vi "Begin.vi"(8 "error in":errorcluster) -> (0 "error out":errorcluster)   [LabVIEW 2015]
doc: "Called before other user functions, this VI is expected to open initial I/O refnums, load in file data, and do all program initialization. Notice that the <B>error out</B> terminal is simply used for data flow. Wiring it to other structures or subVIs ensures that this VI runs first."
uses:
  <vilib>/Rock Robotics/WPI/SafetyOutput/WPI_SafetyOutputConfigMenu.ctl
  <vilib>/Rock Robotics/WPI/DriverStation/WPI_DriverStationRobotMode2.ctl
  <vilib>/Rock Robotics/WPI/Joystick/WPI_JoystickDeviceEnum.ctl
  <vilib>/Rock Robotics/SystemInterfaces/DIO/FPGA_DIOChannel.ctl
  <vilib>/Rock Robotics/SystemInterfaces/DIO/FPGA_DIORelayChannel.ctl
  <vilib>/Rock Robotics/WPI/Solenoid/WPI_SolenoidChannel.ctl
  <vilib>/Rock Robotics/SystemInterfaces/DIO/FPGA_DIOPWMChannel.ctl
  <vilib>/Rock Robotics/SystemInterfaces/spilib/spi_bus.ctl
  Robot Global Data.vi
  <vilib>/Rock Robotics/Network Tables/NT Write String Array.vi
  <vilib>/Rock Robotics/WPI/Switch/WPI_SwitchOpenLimit.vi
  <vilib>/Rock Robotics/WPI/Solenoid/WPI_SolenoidOpenDouble.vi
  <vilib>/Rock Robotics/WPI/Counter/WPI_CounterDigitalInputToDigitalSource.vi
  <vilib>/Rock Robotics/WPI/MotorControl/WPI_MotorControlOpen VictorSP.vi
  <vilib>/Rock Robotics/WPI/MotorControl/WPI_MotorControlOpenCANTalonSRX.vi
  <vilib>/Rock Robotics/WPI/RobotDrive/WPI_RobotDriveOpen4MotorWithExistingMotors.vi
  <vilib>/Rock Robotics/WPI/Gyro/WPI_GyroXRS450_SPI_Open.vi
  <vilib>/Rock Robotics/WPI/Utilities/WPI_GetSetVariantRefNum.vi
  <vilib>/Rock Robotics/WPI/Accelerometer/InternalAccelerometer/WPI_AccelerometerInternalOpen.vi
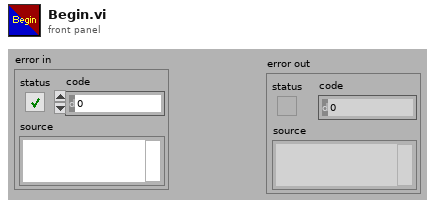
[diagram p1: front panel]
types:
  T1 = typedef "spi_bus.ctl" = enum16{"SPI On-Board, CS0", "SPI On-Board, CS1", "SPI On-Board, CS2", "SPI On-Board, CS3", "SPI MXP", "Invalid"}
  T2 = typedef "FPGA_DIOPWMChannel.ctl" = enum8{"PWM 0", "PWM 1", "PWM 2", "PWM 3", "PWM 4", "PWM 5", "PWM 6", "PWM 7", "PWM 8", "PWM 9", "PWM MXP 0", "PWM MXP 1", "PWM MXP 2", "PWM MXP 3", "PWM MXP 4", "PWM MXP 5", "PWM MXP 6", "PWM MXP 7", "PWM MXP 8", "PWM MXP 9", "Invalid"}
  T3 = typedef "FPGA_DIOChannel.ctl" = enum8{"DIO 0", "DIO 1", "DIO 2", "DIO 3", "DIO 4", "DIO 5", "DIO 6", "DIO 7", "DIO 8", "DIO 9", "DIO MXP 0", "DIO MXP 1", "DIO MXP 2", "DIO MXP 3", "DIO MXP 4", "DIO MXP 5", "DIO MXP 6", "DIO MXP 7", "DIO MXP 8", "DIO MXP 9", "DIO MXP 10", "DIO MXP 11", "DIO MXP 12", "DIO MXP 13", "DIO MXP 14", "DIO MXP 15", "Invalid"}
  T4 = typedef "WPI_SolenoidChannel.ctl" = enum8{"Solenoid 0", "Solenoid 1", "Solenoid 2", "Solenoid 3", "Solenoid 4", "Solenoid 5", "Solenoid 6", "Solenoid 7", "Invalid"}
  T5 = typedef "FPGA_DIORelayChannel.ctl" = enum8{"Relay 0", "Relay 1", "Relay 2", "Relay 3", "Invalid"}
  T6 = typedef "WPI_JoystickDeviceEnum.ctl" = enum16{"USB 0", "USB 1", "USB 2", "USB 3", "USB 4", "USB 5"}
  T7 = typedef "WPI_DriverStationRobotMode2.ctl" = enum16{"Autonomous Disabled", "Autonomous Enabled", "Teleop Disabled", "Teleop Enabled", "Disconnected", "Finish", "Test Disabled", "Test Enabled", "Emergency Stopped"}
  T8 = typedef "WPI_SafetyOutputConfigMenu.ctl" = enum16{"Enable", "Disable"}
  T9 = typedef "WPI_ServoDeviceRef.ctl" = cluster{"DeviceStatus":errorcluster, "PWM Channel":T2, "DeadBand":T10}
  T10 = typedef "WPI_PWMDeadband.ctl" = cluster{"Name":string, "maxPositivePwm":i32, "minPositivePwm":i32, "centerPwm":i32, "maxNegativePwm":i32, "minNegativePwm":i32, "angularRange":u16}
  T11 = typedef "WPI_MotorControlDeviceRef.ctl" = cluster{"DeviceStatus":errorcluster, "Type":T12, "PWM":cluster{"PWM Channel":T2, "DeadBand":T10}, "CAN":cluster{"Device Number":u8, "Control Mode":T13, "Semaphore":T14, "Max Vout":dbl, "TalonSRX Control Mode":T15}, "Invert":bool}
  T12 = typedef "WPI_MotorControlType.ctl" = enum16{"PWM", "CAN", "CANTalonSRX"}
  T13 = typedef "WPI_CANJaguar_ControlMode.ctl" = enum8{"Percent VBus", "Current", "Speed", "Position", "Voltage"}
  T14 = typedef "Semaphore RefNum" = refnum<k1>
  T15 = typedef "WPI_CANTalonSRX_APIControlMode.ctl" = enum8{"Percent VBus", "Speed", "Position", "Slave", "Unchanged / Invalid", "Voltage Compensation", "Current", "Motion Profile"}
  T16 = typedef "WPI_DigitalInputDevRef.ctl" = cluster{"DevStatus":errorcluster, "DIO Channel":T3}
  T17 = typedef "WPI_SolenoidDevRef.ctl" = cluster{"DevStatus":errorcluster, "Pneumatics Control Module":u8, "Forward Solenoid Channel":T4, "Reverse Solenoid Channel":T4}
  T18 = typedef "WPI_JoystickDevRef.ctl" = cluster{"Device":T6}
  T19 = typedef "FPGA_CounterEncoderSourceConvertionLVSourceType.ctl" = cluster{"DevStatus":errorcluster, "AnalogTriggerMode?":bool, "DigitalMode":cluster{"DIO Channel":T20}, "AnalogTriggerMode":cluster{"AnalogTriggerIndex":T21, "OutputType":T22}}
  T20 = typedef "FPGA_DIODigitalSourceChannel.ctl" = enum8{"DIO 0", "DIO 1", "DIO 2", "DIO 3", "DIO 4", "DIO 5", "DIO 6", "DIO 7", "DIO 8", "DIO 9", "DIO MXP 0", "DIO MXP 1", "DIO MXP 2", "DIO MXP 3", "DIO MXP 4", "DIO MXP 5", "DIO MXP 6", "DIO MXP 7", "DIO MXP 8", "DIO MXP 9", "DIO MXP 10", "DIO MXP 11", "DIO MXP 12", "DIO MXP 13", "DIO MXP 14", "DIO MXP 15", "Disabled"}
  T21 = typedef "FPGA_AnalogTriggerIndex.ctl" = enum8{"Trig 0", "Trig 1", "Trig 2", "Trig 3", "Trig 4", "Trig 5", "Trig 6", "Trig 7", "Invalid"}
  T22 = typedef "FPGA_AnalogTriggerOutType.ctl" = enum16{"InWindow", "TriggerState", "Rising", "Falling"}
  T23 = typedef "WPI_EncoderDevRef.ctl" = cluster{"DevStatus":errorcluster, "EncoderIndex":T24, "CounterIndex":T25, "DistancePerCount":dbl, "Decoding Type":T26}
  T24 = typedef "FPGA_EncoderIdx.ctl" = enum8{"Enc 0", "Enc 1", "Enc 2", "Enc 3", "Enc 4", "Enc 5", "Enc 6", "Enc 7", "Invalid"}
  T25 = typedef "FPGA_CounterCtrSystemIndex.ctl" = enum8{"Ctr 0", "Ctr 1", "Ctr 2", "Ctr 3", "Ctr 4", "Ctr 5", "Ctr 6", "Ctr 7", "Invalid"}
  T26 = typedef "WPI_EncoderType.ctl" = enum16{"1x", "2x", "4x"}
  T27 = typedef "WPI_RobotDriveDevRef.ctl" = cluster{"DevStatus":errorcluster, "Motors[]":T11[], "Square Inputs":bool, "Max Output":dbl}
  T28 = typedef "WPI_RelayDevRef.ctl" = cluster{"DevStatus":errorcluster, "Relay Channel":T5, "Relay Direction":T29}
  T29 = typedef "WPI_RelayDirection.ctl" = enum16{"Both directions", "Forward only", "Reverse only"}
  T30 = typedef "WPI_SwitchDevRef.ctl" = cluster{"DevStatus":errorcluster, "DIO Channel":T3, "CntIndex":T25, "Normally Closed":bool}
  T31 = typedef "WPI_AccelerometerDevRef.ctl" = cluster{"DevStatus":errorcluster, "Scaling":T32, "Analog Channels":T33, "I2C Bus":T35, "SPI Bus":T1, "Accel Range":T36, "ADXL Axes":T37, "Handle":i32, "Device Address":u8, "Accel Type":enum16{"Analog", "ADXL345 I2C", "ADXL345 SPI", "Internal", "ADXL362 SPI"}}
  T32 = typedef "WPI_AccelerometerScaling.ctl" = cluster{"Gain (VoltsPerG)":dbl, "Center Voltage":dbl}
  T33 = typedef "WPI_AccelerometerAnalogChannels.ctl" = cluster{"X-Axis":T34, "Y-Axis":T34, "Z-Axis":T34}
  T34 = typedef "FPGA_AIChannel.ctl" = enum8{"AI 0", "AI 1", "AI 2", "AI 3", "AI MXP 0", "AI MXP 1", "AI MXP 2", "AI MXP 3", "Invalid"}
  T35 = typedef "i2c_bus.ctl" = enum16{"I2C On-Board", "I2C MXP", "Invalid"}
  T36 = typedef "ADXL345 Range.ctl" = u8
  T37 = typedef "WPI_AccelerometerADXL345 Axes.ctl" = cluster{"X-Axis":bool, "Y-Axis":bool, "Z-Axis":bool}
  T38 = typedef "WPI_GyroDevRef.ctl" = cluster{"DevStatus":errorcluster, "Analog Channel":T34, "Offset":dbl, "Gain (VoltsPerDegree/Second)":dbl, "Gyro Type":enum16{"Analog", "XRS450"}, "Handle":i32, "SPI Bus":T1, "Device Found":bool, "Sample Rate":dbl, "Calibrate On Open":bool}
  T39 = typedef "WPI_CompressorDevRef.ctl" = cluster{"DevStatus":errorcluster, "Pneumatics Control Module":u8}
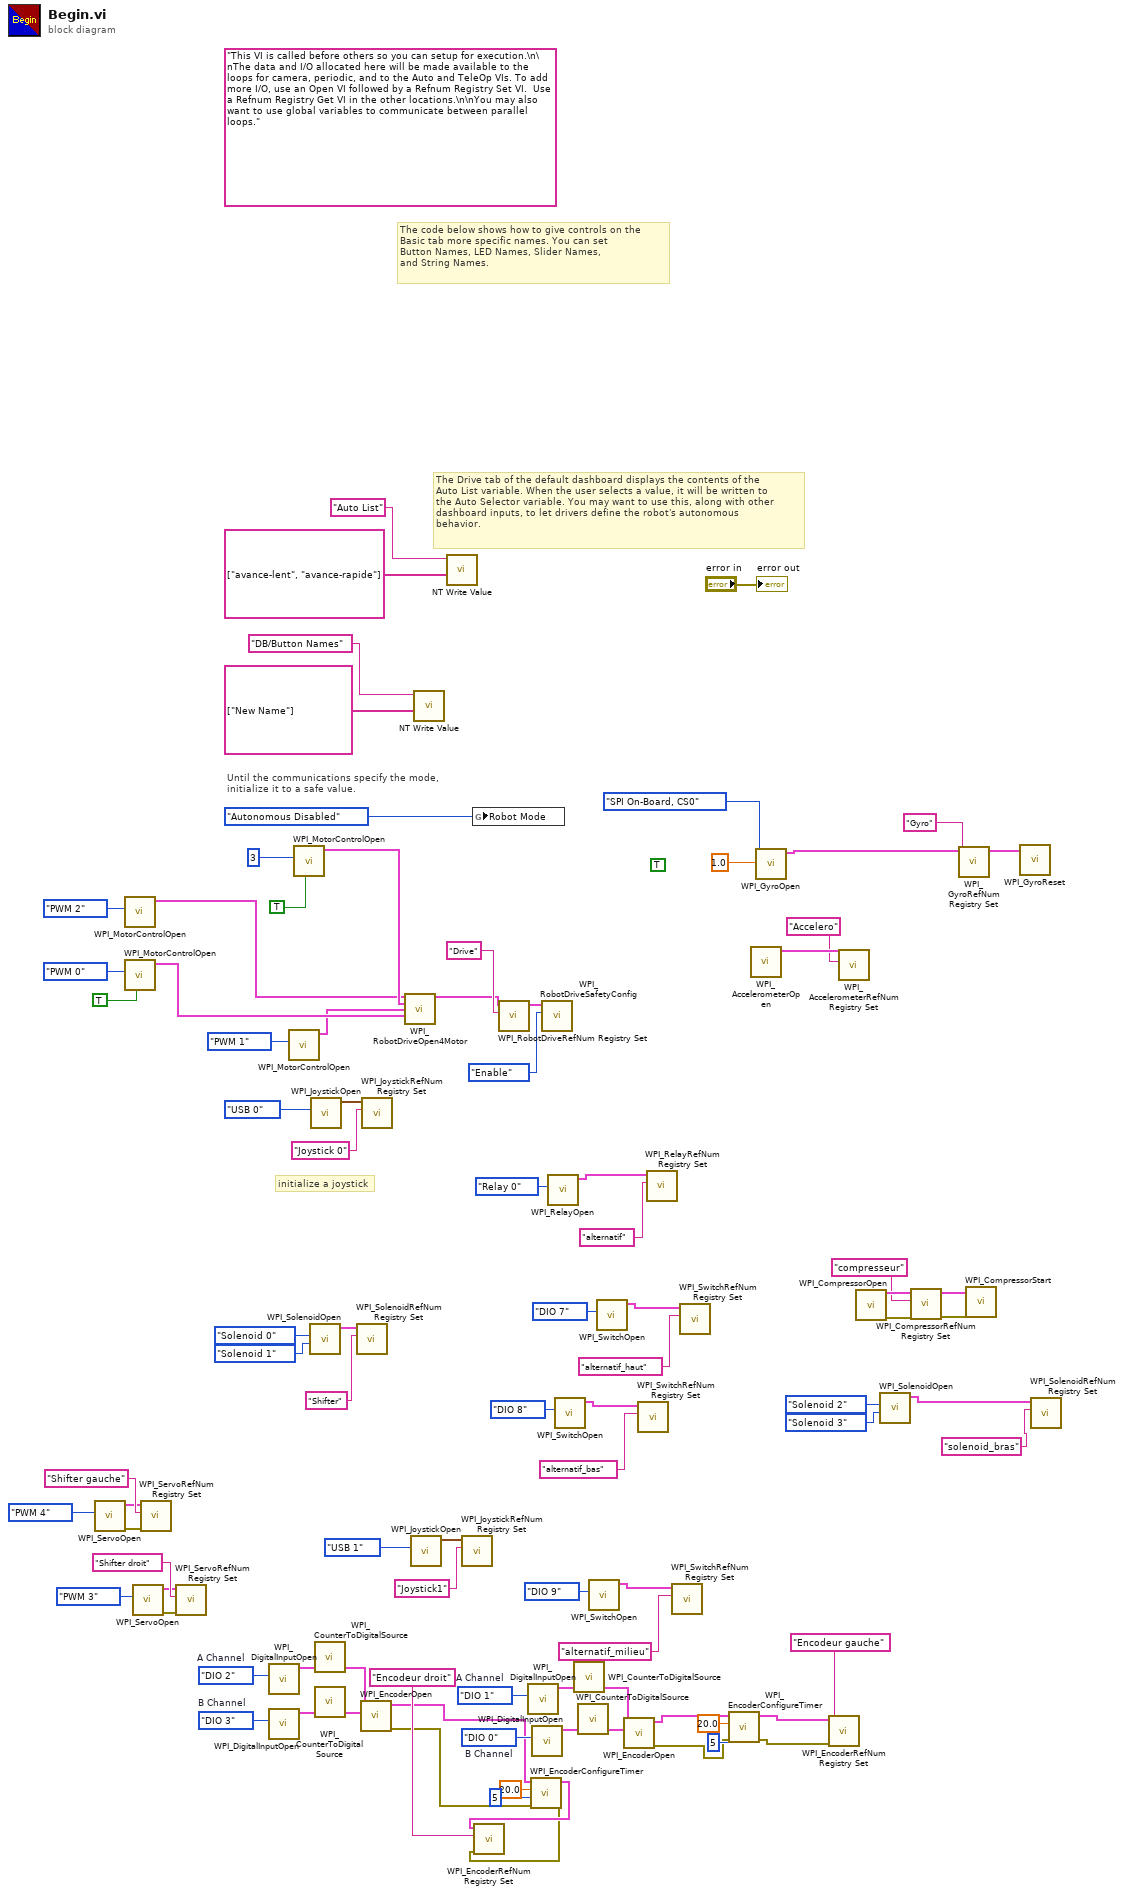
[diagram p0: block diagram]
diagram:
  (unwired) TRUE ("Calibrate On Open")
  w37 = FPGA_DIOChannel."DIO 0"  # B Channel
  w36 = FPGA_DIOChannel."DIO 1"  # A Channel
  w44 = FPGA_DIOChannel."DIO 3"  # B Channel
  w43 = FPGA_DIOChannel."DIO 2"  # A Channel
  (unwired) "This VI is called before others so you can setup for execution.\n\nThe data and I/O allocated here will be made available to the loops for camera, periodic, and to the Auto and TeleOp VIs. To add more I/O, use an Open VI followed by a Refnum Registry Set VI.  Use a Refnum Registry Get VI in the other locations.\n\nYou may also want to use global variables to communicate between parallel loops."
  # "The Drive tab of the default dashboard displays the contents of the\nAuto List variable. When the user selects a value, it will be written to\nthe Auto Selector variable. You may want to use this, along with other\ndashboard inputs, to let drivers define the robot's autonomous\nbehavior."
  # "The code below shows how to give controls on the\nBasic tab more specific names. You can set\nButton Names, LED Names, Slider Names,\nand String Names."
  # "initialize a joystick"
  # "Until the communications specify the mode,\ninitialize it to a safe value."
  n1 = call <vilib>:"WPI_ServoOpen.vi"("PWM Channel"=FPGA_DIOPWMChannel."PWM 4" ("Front Left Motor")) -> ("error out"=w48:errorcluster, "ServoDeviceRef"=w49:T9)  [unwired: 9 in]
  n2 = call-poly <vilib>:"WPI_MotorControlOpen.vi"("PWM Channel"=FPGA_DIOPWMChannel."PWM 2") -> ("MotorControlDeviceRef"=w22:T11)  [unwired: 9 in, 1 out]
  n3 = call-poly <vilib>:"WPI_MotorControlOpen.vi"("Invert"=TRUE, "PWM Channel"=FPGA_DIOPWMChannel."PWM 0") -> ("MotorControlDeviceRef"=w21:T11)  [unwired: 8 in, 1 out]
  n4 = call <vilib>:"WPI_ServoOpen.vi"("PWM Channel"=FPGA_DIOPWMChannel."PWM 3" ("Front Left Motor")) -> ("error out"=w47:errorcluster, "ServoDeviceRef"=w50:T9)  [unwired: 9 in]
  n5 = call <vilib>:"WPI_ServoRefNum Registry Set.vi"("error in (no error)"=w48, "refnum name"="Shifter gauche", "ServoDeviceRef"=w49) -> ()  [unwired: 7 in, 2 out]
  n6 = call <vilib>:"WPI_ServoRefNum Registry Set.vi"("error in (no error)"=w47, "refnum name"="Shifter droit", "ServoDeviceRef"=w50) -> ()  [unwired: 7 in, 2 out]
  n7 = call <vilib>:"WPI_DigitalInputOpen.vi"("DIO Channel"=w43) -> ("DigitalInputDevRef"=w40:T16)  [unwired: 1 in, 9 out]
  n8 = call <vilib>:"WPI_DigitalInputOpen.vi"("DIO Channel"=w44) -> ("DigitalInputDevRef"=w41:T16)  [unwired: 1 in, 9 out]
  n9 = call-poly <vilib>:"WPI_MotorControlOpen.vi"("PWM Channel"=FPGA_DIOPWMChannel."PWM 1") -> ("MotorControlDeviceRef"=w20:T11)  [unwired: 9 in, 1 out]
  n10 = call-poly <vilib>:"WPI_MotorControlOpen.vi"("Invert"=TRUE, "Device Number"=u8 3) -> ("MotorControlDeviceRef"=w23:T11)  [unwired: 8 in, 1 out]
  n11 = call-poly <vilib>:"WPI_SolenoidOpen.vi"("Reverse Solenoid Channel"=WPI_SolenoidChannel."Solenoid 1", "Forward Solenoid Channel"=WPI_SolenoidChannel."Solenoid 0") -> ("SolenoidDevRef"=w60:T17)  [unwired: 8 in, 1 out]
  n12 = call <vilib>:"WPI_JoystickOpen.vi"("JoystickDevice"=WPI_JoystickDeviceEnum."USB 0") -> ("JoystickDevRef"=w87:T18)  [unwired: 10 in]
  n13 = call-poly <vilib>:"WPI_CounterToDigitalSource.vi"("DigitalInputDevRef"=w40) -> ("Digital Source"=w39:T19)  [unwired: 6 out]
  n14 = call-poly <vilib>:"WPI_CounterToDigitalSource.vi"("DigitalInputDevRef"=w41) -> ("Digital Source"=w42:T19)  [unwired: 6 out]
  n15 = call <vilib>:"WPI_SolenoidRefNum Registry Set.vi"("refnum name"="Shifter", "SolenoidDevRef"=w60) -> ()  [unwired: 8 in, 2 out]
  n16 = call <vilib>:"WPI_EncoderOpen.vi"("BSource"=w42, "ASource"=w39) -> ("error out"=w4:errorcluster, "EncoderDevRef"=w6:T23)  [unwired: 6 in, 2 out]
  n17 = call <vilib>:"WPI_JoystickRefNum Registry Set.vi"("refnum name"="Joystick 0", "JoystickDevRef"=w87) -> ()  [unwired: 8 in, 2 out]
  n18 = call-poly <vilib>:"WPI_RobotDriveOpen4Motor.vi"("Rear Left Motor Dev Ref"=w22, "Rear Right Motor Dev Ref"=w23, "Front Left Motor Dev Ref"=w20, "Front Right Motor Dev Ref"=w21) -> ("RobotDriveDevRef"=w26:T27)  [unwired: 10 in, 1 out]
  n19 = call <vilib>:"WPI_JoystickOpen.vi"("JoystickDevice"=WPI_JoystickDeviceEnum."USB 1") -> ("JoystickDevRef"=w71:T18)  [unwired: 10 in]
  n20 = call-poly <vilib>:"NT Write Value.vi"("String Array"=string[] ["New Name"], "Name"="DB/Button Names") -> ()  [unwired: 9 in, 1 out]
  n21 = call-poly <vilib>:"NT Write Value.vi"("String Array"=string[] ["avance-lent", "avance-rapide"], "Name"="Auto List") -> ()  [unwired: 9 in, 1 out]
  n22 = call <vilib>:"WPI_JoystickRefNum Registry Set.vi"("refnum name"="Joystick1", "JoystickDevRef"=w71) -> ()  [unwired: 8 in, 2 out]
  n23 = global write "Robot Global Data.vi" "Robot Mode"(WPI_DriverStationRobotMode2."Autonomous Disabled" ("Robot Mode")) -> ()
  n24 = call <vilib>:"WPI_RobotDriveRefNum Registry Set.vi"("refnum name"="Drive", "RobotDriveDevRef"=w26) -> ("RobotDriveDevRef"=w91:T27)  [unwired: 2 in, 7 out]
  n25 = call <vilib>:"WPI_DigitalInputOpen.vi"("DIO Channel"=w36) -> ("DigitalInputDevRef"=w33:T16)  [unwired: 1 in, 9 out]
  n26 = call <vilib>:"WPI_EncoderConfigureTimer.vi"("error in (no error)"=w4, "Number Samples to Average"=u8 5, "Minimum Rate"=20.0, "EncoderDevRef"=w6) -> ("error out"=w3:errorcluster, "EncoderDevRef"=w5:T23)  [unwired: 6 in]
  n27 = call <vilib>:"WPI_EncoderRefNum Registry Set.vi"("error in (no error)"=w3, "refnum name"="Encodeur droit", "EncoderDevRef"=w5) -> ()  [unwired: 7 in, 2 out]
  n28 = call <vilib>:"WPI_DigitalInputOpen.vi"("DIO Channel"=w37) -> ("DigitalInputDevRef"=w34:T16)  [unwired: 1 in, 9 out]
  n29 = call <vilib>:"WPI_RobotDriveSafetyConfig.vi"("mode"=WPI_SafetyOutputConfigMenu."Enable", "RobotDriveDevRef"=w91) -> ()  [unwired: 8 in, 2 out]
  n30 = call <vilib>:"WPI_RelayOpen.vi"("Relay Channel"=FPGA_DIORelayChannel."Relay 0") -> ("RelayDevRef"=w66:T28)  [unwired: 9 in, 1 out]
  n31 = call-poly <vilib>:"WPI_SwitchOpen.vi"("DIO Channel"=FPGA_DIOChannel."DIO 8") -> ("SwitchDevRef"=w74:T30)  [unwired: 9 in, 1 out]
  n32 = call-poly <vilib>:"WPI_CounterToDigitalSource.vi"("DigitalInputDevRef"=w33) -> ("Digital Source"=w32:T19)  [unwired: 6 out]
  n33 = call-poly <vilib>:"WPI_CounterToDigitalSource.vi"("DigitalInputDevRef"=w34) -> ("Digital Source"=w35:T19)  [unwired: 6 out]
  n34 = call-poly <vilib>:"WPI_SwitchOpen.vi"("DIO Channel"=FPGA_DIOChannel."DIO 9") -> ("SwitchDevRef"=w67:T30)  [unwired: 9 in, 1 out]
  n35 = call-poly <vilib>:"WPI_SwitchOpen.vi"("DIO Channel"=FPGA_DIOChannel."DIO 7") -> ("SwitchDevRef"=w77:T30)  [unwired: 9 in, 1 out]
  n36 = call <vilib>:"WPI_EncoderOpen.vi"("BSource"=w35, "ASource"=w32) -> ("error out"=w7:errorcluster, "EncoderDevRef"=w12:T23)  [unwired: 6 in, 2 out]
  n37 = call <vilib>:"WPI_SwitchRefNum Registry Set.vi"("refnum name"="alternatif_bas", "SwitchDevRef"=w74) -> ()  [unwired: 8 in, 2 out]
  n38 = call <vilib>:"WPI_RelayRefNum Registry Set.vi"("refnum name"="alternatif", "RelayDevRef"=w66) -> ()  [unwired: 8 in, 2 out]
  n39 = call <vilib>:"WPI_SwitchRefNum Registry Set.vi"("refnum name"="alternatif_milieu", "SwitchDevRef"=w67) -> ()  [unwired: 8 in, 2 out]
  n40 = call <vilib>:"WPI_SwitchRefNum Registry Set.vi"("refnum name"="alternatif_haut", "SwitchDevRef"=w77) -> ()  [unwired: 8 in, 2 out]
  n41 = call <vilib>:"WPI_EncoderConfigureTimer.vi"("error in (no error)"=w7, "Number Samples to Average"=u8 5, "Minimum Rate"=20.0, "EncoderDevRef"=w12) -> ("error out"=w8:errorcluster, "EncoderDevRef"=w11:T23)  [unwired: 6 in]
  n42 = call-poly <vilib>:"WPI_AccelerometerOpen.vi"() -> ("AccelerometerDevRef"=w14:T31)  [unwired: 10 in, 1 out]
  n43 = call-poly <vilib>:"WPI_GyroOpen.vi"("Sample Rate (ms)"=1.0, "SPI Bus"=spi_bus."SPI On-Board, CS0") -> ("GyroDevRef"=w25:T38)  [unwired: 8 in, 1 out]
  n44 = call <vilib>:"WPI_EncoderRefNum Registry Set.vi"("error in (no error)"=w8, "refnum name"="Encodeur gauche", "EncoderDevRef"=w11) -> ()  [unwired: 7 in, 2 out]
  n45 = call <vilib>:"WPI_AccelerometerRefNum Registry Set.vi"("refnum name"="Accelero", "AccelerometerDevRef"=w14) -> ()  [unwired: 8 in, 2 out]
  n46 = call <vilib>:"WPI_CompressorOpen.vi"() -> ("CompressorDevRef"=w56:T39, "error out"=w57:errorcluster)  [unwired: 14 in]
  n47 = call-poly <vilib>:"WPI_SolenoidOpen.vi"("Reverse Solenoid Channel"=WPI_SolenoidChannel."Solenoid 3", "Forward Solenoid Channel"=WPI_SolenoidChannel."Solenoid 2") -> ("SolenoidDevRef"=w64:T17)  [unwired: 8 in, 1 out]
  n48 = call <vilib>:"WPI_CompressorRefNum Registry Set.vi"("error in (no error)"=w57, "refnum name"="compresseur", "CompressorDevRef"=w56) -> ("error out"=w53:errorcluster, "CompressorDevRef"=w55:T39)  [unwired: 7 in]
  n49 = call <vilib>:"WPI_GyroRefNum Registry Set.vi"("refnum name"="Gyro", "GyroDevRef"=w25) -> ("GyroDevRef"=w15:T38)  [unwired: 8 in, 1 out]
  n50 = call <vilib>:"WPI_CompressorStart.vi"("error in (no error)"=w53, "CompressorDevRef"=w55) -> ()  [unwired: 8 in, 2 out]
  n51 = call <vilib>:"WPI_GyroReset.vi"("GyroDevRef"=w15) -> ()  [unwired: 9 in, 2 out]
  n52 = call <vilib>:"WPI_SolenoidRefNum Registry Set.vi"("refnum name"="solenoid_bras", "SolenoidDevRef"=w64) -> ()  [unwired: 8 in, 2 out]
  "error out" <- "error in"
